vi "AudioTest.Inc Dec UUT Dir.vi"(9 "Increment":bool, 10 "UUT Dir Order":enum16{"Name", "Date"}(ring), 11 "SoundCheck Data File":path caption="Data File") -> (1 "FolderNavStatus":T1, 3 "Next Folder":path)   [LabVIEW 2018]
uses:
  TypeDefs/AudioTest.Analysis Folder Navigation Status.ctl
  <vilib>/KATE/Files/File Utils.lvlib
panel:
  out "Index":i32
  in  "Test":bool
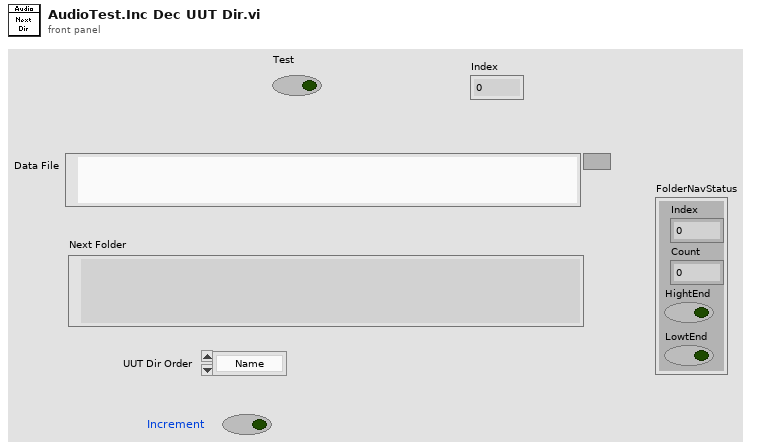
[diagram p1: front panel]
types:
  T1 = typedef "AudioTest.Analysis Folder Navigation Status.ctl" = cluster{"Index":i32, "Count":i32, "HightEnd":bool, "LowtEnd":bool}
  T2 = cluster{"last mod":timestamp, "appended path":path}
  T3 = cluster{"last mod":timestamp, "appended path":path}[]
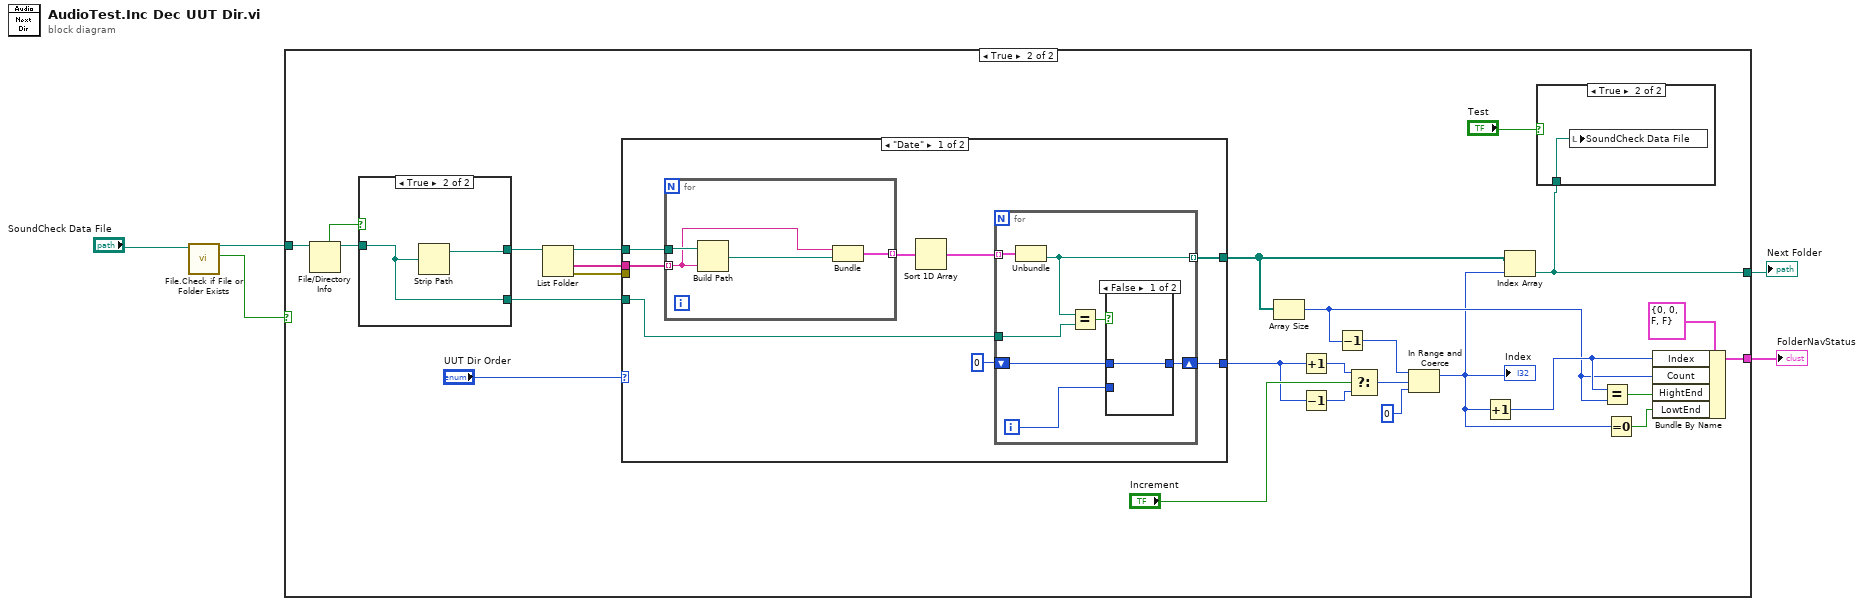
[diagram p0: block diagram]
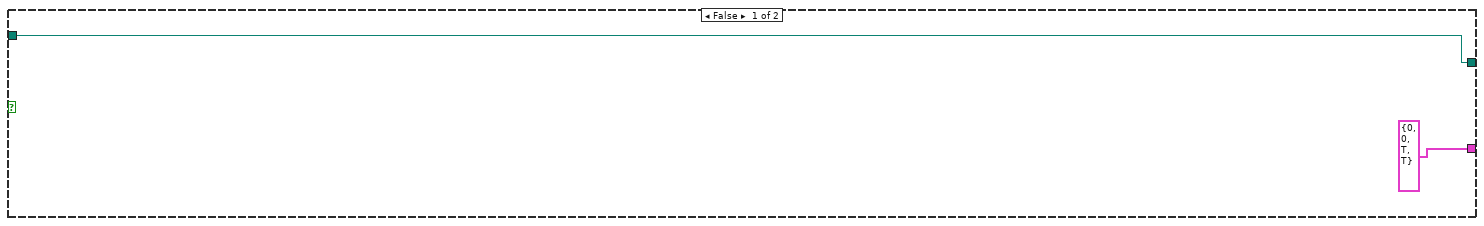
[diagram p2: hidden frame]
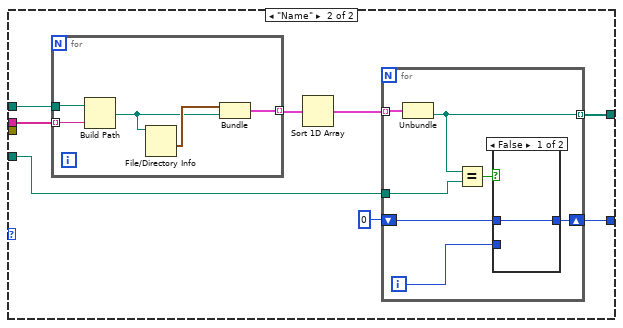
[diagram p5: hidden frame]
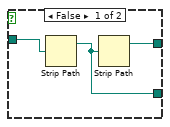
[diagram p7: hidden frame]
diagram:
  n1 = call <vilib>:"File.Check if File or Folder Exists.vi"("Path"="SoundCheck Data File") -> ("Exists"=w2:bool, "Dup Path"=w4:path)  [unwired: 6 in, 3 out]
  n2 = case shown="True" w2 {
    tunnel: w4 -> [w7 w33]
    tunnel: [w7 w15] -> w3
    tunnel: [T1 {"Index"=0, "Count"=0, "HightEnd"=TRUE, "LowtEnd"=TRUE} ("FolderNavStatus") w13] -> w1
    frame False {
    }
    frame True {
      n3 = File/Directory Info(path=w33) -> (path out=w31:path, directory=w32:bool)  [unwired: 1 in, 5 out]
      n4 = case shown="True" w32 {
        tunnel: w31 -> [w80 w81]
        tunnel: [w79 w82] -> w30
        tunnel: [w78 w81] -> w26
        frame False {
          n5 = Strip Path(path=w80) -> (stripped path=w78:path)  [unwired: 1 out]
          n6 = Strip Path(path=w78) -> (stripped path=w79:path)  [unwired: 1 out]
        }
        frame True {
          n7 = Strip Path(path=w81) -> (stripped path=w82:path)  [unwired: 1 out]
        }
      }
      n8 = List Folder(path=w30) -> (path out=w29:path, folder names=w28:string[], error out=w16:errorcluster)  [unwired: 3 in, 1 out]
      n9 = case shown="\"Date\"" "UUT Dir Order" {
        tunnel: w29 -> [w42 w63]
        tunnel: w28 -> [w41 w62]
        tunnel: w26 -> [w38 w59]
        tunnel: [w36 w57] -> w22
        tunnel: [w35 w56] -> w18
        tunnel: w16 -> [_ _]
        frame "Date" {
          n10 = for {
            tunnel: w42 -> [w55]
            tunnel: w41 -> [w52] mode=indexing
            tunnel: [w54] -> w40 mode=indexing
            n11 = Build Path(base path=w55, name or relative path=w52) -> (appended path=w53:path)
            n12 = Bundle(w52, "appended path"=w53) -> (w54:cluster{string, "appended path":path})  [unwired: 1 in]
          }
          n13 = Sort 1D Array(array=w40) -> (sorted array=w39:cluster{string, "appended path":path}[])
          n14 = for {
            tunnel: w39 -> [w49] mode=indexing
            tunnel: [w48] -> w35 mode=indexing
            tunnel: w38 -> [w47]
            shift-right: [w43] -> w36
            shift-left: 0 -> [w45]
            i -> [w44]
            n15 = Unbundle(w49) -> ("appended path"=w48:path)  [unwired: 1 out]
            n16 = Equal?(x=w48, y=w47) -> (x = y?=w46:bool)
            n17 = case shown="False" w46 {
              tunnel: w45 -> [w50 _]
              tunnel: w44 -> [_ w51]
              tunnel: [w50 w51] -> w43
              frame False {
              }
              frame True {
              }
            }
          }
        }
        frame "Name" {
          n18 = for {
            tunnel: w63 -> [w77]
            tunnel: w62 -> [w73] mode=indexing
            tunnel: [w75] -> w61 mode=indexing
            n19 = Build Path(base path=w77, name or relative path=w73) -> (appended path=w74:path)
            n20 = File/Directory Info(path=w74) -> (last mod=w76:timestamp)  [unwired: 1 in, 6 out]
            n21 = Bundle("last mod"=w76, "appended path"=w74) -> (w75:T2)  [unwired: 1 in]
          }
          n22 = Sort 1D Array(array=w61) -> (sorted array=w60:T3)
          n23 = for {
            tunnel: w60 -> [w70] mode=indexing
            tunnel: [w69] -> w56 mode=indexing
            tunnel: w59 -> [w68]
            shift-right: [w64] -> w57
            shift-left: 0 -> [w66]
            i -> [w65]
            n24 = Unbundle(w70) -> ("appended path"=w69:path)  [unwired: 1 out]
            n25 = Equal?(x=w69, y=w68) -> (x = y?=w67:bool)
            n26 = case shown="False" w67 {
              tunnel: w66 -> [w71 _]
              tunnel: w65 -> [_ w72]
              tunnel: [w71 w72] -> w64
              frame False {
              }
              frame True {
              }
            }
          }
        }
      }
      n27 = Array Size(array=w18) -> (size(s)=w10:i32)
      n28 = Increment(x=w22) -> (x+1=w25:i32)
      n29 = Decrement(x=w22) -> (x-1=w24:i32)
      n30 = Decrement(x=w10) -> (x-1=w19:i32)
      n31 = Select(t=w25, s="Increment", f=w24) -> (s? t:f=w21:i32)
      n32 = In Range and Coerce(upper limit=w19, x=w21, lower limit=0) -> (coerced(x)=w8:i32)  [unwired: 1 out]
      "Index" <- w8
      n33 = Increment(x=w8) -> (x+1=w11:i32)
      n34 = Index Array(array=w18, index=w8) -> (element=w15:path)
      n35 = case shown="True" "Test" {
        tunnel: w15 -> [_ w34]
        frame False {
        }
        frame True {
          n36 = local write "SoundCheck Data File"(w34) -> ()
        }
      }
      n37 = Equal?(x=w11, y=w10) -> (x = y?=w12:bool)
      n38 = Equal To 0?(x=w8) -> (x = 0?=w9:bool)
      n39 = Bundle By Name(cluster=T1 {"Index"=0, "Count"=0, "HightEnd"=FALSE, "LowtEnd"=FALSE} ("FolderNavStatus"), "Index"=w11, "Count"=w10, "HightEnd"=w12, "LowtEnd"=w9) -> (w13:T1)
    }
  }
  "Next Folder" <- w3
  "FolderNavStatus" <- w1
